vi "Strafe Correction TF.vi"() -> ()   [LabVIEW 2018]
panel:
  in  "Strafe Correction TF":bool
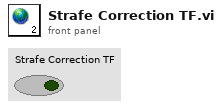
[diagram p1: front panel]
diagram:
